vi "Shooter Ticks.vi"(11 "limelight":dbl) -> (3 "ticks":dbl)   [LabVIEW 2019]
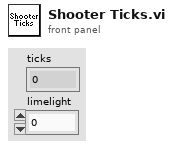
[diagram p1: front panel]
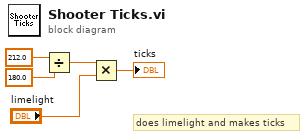
[diagram p0: block diagram]
diagram:
  # "does limelight and makes ticks"
  n1 = Divide(x=212.0, y=180.0) -> (x/y=w4:dbl)
  n2 = Multiply(x=w4, y="limelight") -> (x*y=→"ticks":dbl)
